vi "FPGA_ADC_read_fastseq.vi"(2 "Readout parameter":T2, 3 "FPGA In":T1) -> (0 "data out":dbl[][](array[numeric]), 1 "FPGA Out":T1)   [LabVIEW 2013]
uses:
  fpga-bitfile-ref.ctl
  <vilib>/rvi/interface/common/niFpgaWaitOnOcc.vi
  <vilib>/Utility/error.llb/Error Cluster From Error Code.vi
  <vilib>/rvi/errors/niLvFpgaAdjustHostInterfaceError.vi
  <vilib>/rvi/interface/nirviMethod/nirviMethod.xnode
  FPGA Bitfiles/fpgabatch18_sbRIO9612RIO0_FPGAMAINlock-in_BbNldMosBaM.lvbitx
  <vilib>/FPGAPlugInAG/sbRIO-9612/niLvFpga_ReadFifo_sbRIO-9612.vi
  <vilib>/rvi/errors/niLvFpgaMergeErrorWithErrorCode.vi
panel:
  in  "stop read":bool
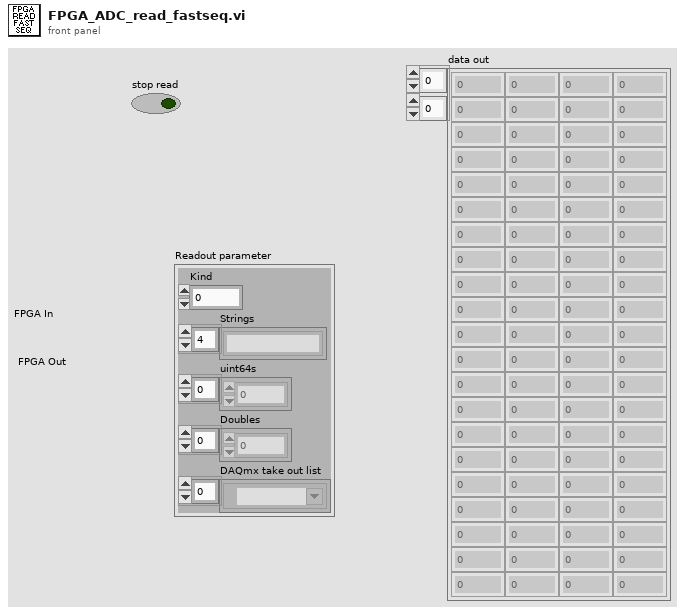
[diagram p1: front panel]
types:
  T1 = typedef "fpga-bitfile-ref.ctl" = refnum<k20>
  T2 = cluster{"Kind":u16, "Strings":string[], "uint64s":u64[], "Doubles":dbl[], "DAQmx take out list":refnum<k21>[]}
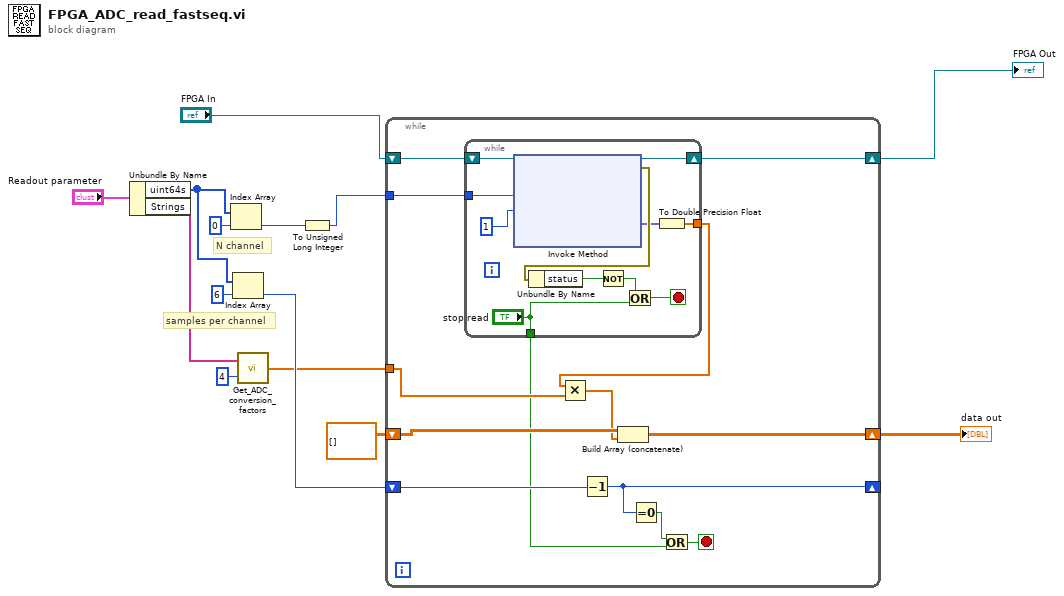
[diagram p0: block diagram]
diagram:
  # "samples per channel"
  # "N channel"
  n1 = Unbundle By Name("Readout parameter") -> ("uint64s"=w10:u64[], "Strings"=w7:string[])
  n2 = Index Array(array=w10, index=0) -> (element=w12:u64)
  n3 = Index Array(array=w10, index=6) -> (element=w9:u64)
  n4 = call "Get_ADC_conversion_factors.vi"("index"=4, "Strings"=w7) -> ("elements"=w6:dbl[])
  n5 = To Unsigned Long Integer(number=w12) -> (unsigned 32bit integer=w3:u32)
  n6 = while {
    shift-right: [w24] -> w5
    shift-left: dbl[][] [] -> [w27]
    shift-right: [w25] -> w4
    shift-left: "FPGA In" -> [w26]
    tunnel: w3 -> [w23]
    shift-right: [w15] -> _
    shift-left: w9 -> [w19]
    tunnel: w6 -> [w21]
    stop <- w16 stop-if-true
    n7 = while {
      tunnel: [w31] -> w22
      shift-right: [w37] -> w25
      shift-left: w26 -> [w32]
      tunnel: w23 -> [w29]
      tunnel: ["stop read"] -> w18
      stop <- w33 stop-if-true
      n8 = xnode "Invoke Method"("FPGA VI Reference In"=w32, "Number of Elements"=w29, "Timeout (ms)"=1) -> ("FPGA VI Reference Out"=w37:T1, "error out"=w36:errorcluster, "Data"=w30:fxp<+/-,26,5>[])  [unwired: 1 in, 1 out]
      n9 = Unbundle By Name(w36) -> ("status"=w35:bool)
      n10 = Not(x=w35) -> (.not. x?=w34:bool)
      n11 = Or(x=w34, y="stop read") -> (x .or. y?=w33:bool)
      n12 = To Double Precision Float(number=w30) -> (double precision float=w31:dbl[])
    }
    n13 = Multiply(x=w22, y=w21) -> (x*y=w20:dbl[])
    n14 = Decrement(x=w19) -> (x-1=w15:u64)
    n15 = Build Array (concatenate)(w27, w20) -> (w24:dbl[][])
    n16 = Equal To 0?(x=w15) -> (x = 0?=w17:bool)
    n17 = Or(x=w17, y=w18) -> (x .or. y?=w16:bool)
  }
  "FPGA Out" <- w4
  "data out" <- w5
